vi "ReadCapacity.vi"(11 "TypedCircularBuffer in":refnum<class "RefTypedCircularBuffer.lvclass">) -> (2 "capacity":u32, 3 "TypedCircularBuffer out":refnum<class "RefTypedCircularBuffer.lvclass">)   [LabVIEW 2024, in "RefTypedCircularBuffer.lvclass"]
uses:
  RefTypedCircularBuffer.lvclass
  RefTypedCircularBuffer.lvclass/RefTypedCircularBuffer.ctl
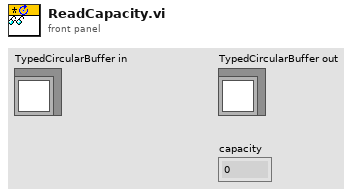
[diagram p1: front panel]
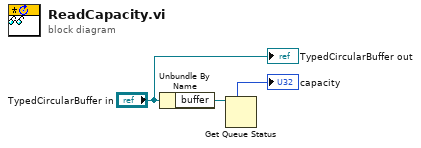
[diagram p0: block diagram]
diagram:
  n1 = Unbundle By Name("TypedCircularBuffer in") -> ("buffer"=w2:refnum<queue>)
  n2 = Get Queue Status(queue=w2) -> (max queue size=→"capacity":i32)  [unwired: 2 in, 7 out]
  "TypedCircularBuffer out" <- "TypedCircularBuffer in"
